vi "Davies_Bouldin_Score.vi"(8 "error in (no error)":errorcluster caption="entrée d'erreur (pas d'erreur)", 10 "labels":string[][](array[string]), 11 "X":string[][](array[string])) -> (0 "error out":errorcluster caption="sortie d'erreur", 3 "Score":string)   [LabVIEW 2020]
doc: "Computes the Davies-Bouldin score.\n\nThe score is defined as the average similarity measure of each cluster with its most similar cluster, where similarity is the ratio of within-cluster distances to between-cluster distances. Thus, clusters which are farther apart and less dispersed will result in a better score.\n\nThe minimum score is zero, with lower values indicating better clustering.\n\n\n\nParameters :\n\n- X : array-like, shape (n_samples, n_features)\nList of n_features-dimensional data points. Each row corresponds to a single data point.\n\n- labels : array-like, shape (n_samples,)\nPredicted labels for each sample.\n\nReturns : \n\n- score : float\nThe resulting Davies-Bouldin score."
uses:
  Davies_Bouldin_Score.lvclass
panel:
  out "Davies_Bouldin_Score.lvclass":refnum<class "Davies_Bouldin_Score.lvclass">
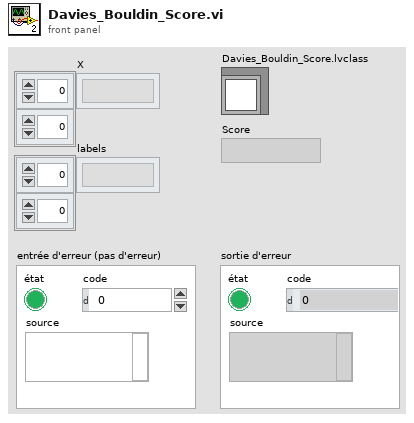
[diagram p1: front panel]
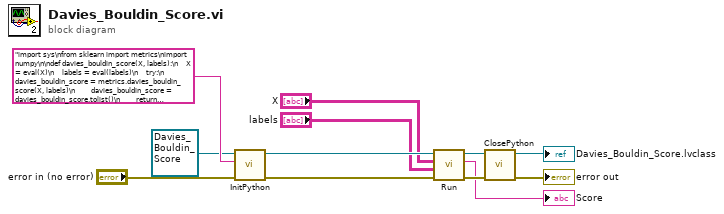
[diagram p0: block diagram]
diagram:
  n1 = call-dynamic "InitPython.vi"("error in (no error)"="error in (no error)", "Python Instruction"="import sys\nfrom sklearn import metrics\nimport numpy\n\ndef davies_bouldin_score(X, labels):\n    X = eval(X)\n    labels = eval(labels)\n    try:\n        davies_bouldin_score = metrics.davies_bouldin_score(X, labels)\n        davies_bouldin_score = davies_bouldin_score.tolist()\n        return str(davies_bouldin_score)\n    except:\n        erreur = sys.exc_info()\n        typerr = u\"%s\" % (erreur[0])\n        typerr = typerr[typerr.find(\"'\")+1:typerr.rfind(\"'\")]\n        msgerr = u\"%s\" % (erreur[1])\n        message = str('/!\\\\ {0} : {1}'. format(typerr,msgerr))\n        return message", "Scikit-learn en entrée"=refnum<class "Davies_Bouldin_Score.lvclass"> refnum ("Davies_Bouldin_Score.lvclass")) -> ("error out"=w5:errorcluster, "Scikit-learn en sortie"=w9:refnum<class "Davies_Bouldin_Score.lvclass">)  [unwired: 7 in]
  n2 = call-dynamic "Run.vi"("error in (no error)"=w5, "labels"="labels", "X"="X", "Davies_Bouldin_Score.lvclass"=w9) -> ("error out"=w7:errorcluster, "Score"=→"Score":string, "Davies_Bouldin_Score.lvclass"=w8:refnum<class "Davies_Bouldin_Score.lvclass">)  [unwired: 5 in]
  n3 = call-dynamic "ClosePython.vi"("error in (no error)"=w7, "Scikit-learn en entrée"=w8) -> ("error out"=→"error out":errorcluster, "Scikit-learn en sortie"=→"Davies_Bouldin_Score.lvclass":refnum<class "Davies_Bouldin_Score.lvclass">)  [unwired: 8 in]
